vi "Configure FFT.vi"(7 "FFT Parameters":T2={"Direction"=TRUE, "scale_sch"=85.0, "Flush Length"=1500} {"scale_sch" format="%.0b"}, 8 "error in":errorcluster, 11 "FPGA Session":T1) -> (0 "error out":errorcluster, 3 "FPGA Session":T1)   [LabVIEW 2010]
doc: "This VI configures FFT Length, Scaling Parameters from the Host.\n\nThis VI also starts FFT Core on the FPGA and waits for valid input to start processing data."
uses:
  Session/Session Handle.ctl
  FFT Block/FFT/Controls/FFT Parameters.ctl
  <vilib>/rvi/interface/nirviReadWriteControl/nirviReadWriteControl.xnode
  System Integration Test Bench/tb_Interpolate and FFT Loop/tb_interpolation_fft_simio_fpga.vi
  FFT Block/FFT/Controls/FFT States.ctl
  <vilib>/RVI Host/nirviSupport.llb/nirviErrorClusterFromErrorCode.vi
  <vilib>/rvi/errors/niLvFpgaWhatHappensToTopLevelVI.ctl
  <vilib>/rvi/interface/common/niFpgaNodeNameForErrorReporting.ctl
  <vilib>/rvi/errors/niLvFpgaAdjustHostInterfaceError.vi
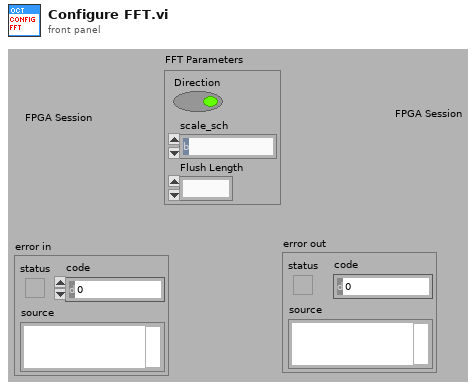
[diagram p1: front panel]
types:
  T1 = typedef "Session Handle.ctl" = refnum<k20>
  T2 = typedef "FFT Parameters.ctl" = cluster{"Direction":bool, "scale_sch":fxp<+,10,10>, "Flush Length":u16}
  T3 = typedef "FFT States.ctl" = enum8{"Configure", "Start FFT processing", "Process", "Unload Last FFT", "Reset"}
  T4 = typedef "niFpgaNodeNameForErrorReporting.ctl" = enum16{"Open FPGA VI Reference", "Read/Write Control", "Invoke Method: Abort", "Invoke Method: Acknowledge IRQ", "Invoke Method: Download", "Invoke Method: FIFO.Configure", "Invoke Method: FIFO.Read", "Invoke Method: FIFO.Start", "Invoke Method: FIFO.Stop", "Invoke Method: FIFO.Write", "Invoke Method: Reset", "Invoke Method: Run", "Invoke Method: Wait on IRQ", "Close FPGA VI Reference"}
  T5 = typedef "niLvFpgaWhatHappensToTopLevelVI.ctl" = enum16{"top level VI scripted behind XNode", "top level VI inlined behind XNode"}
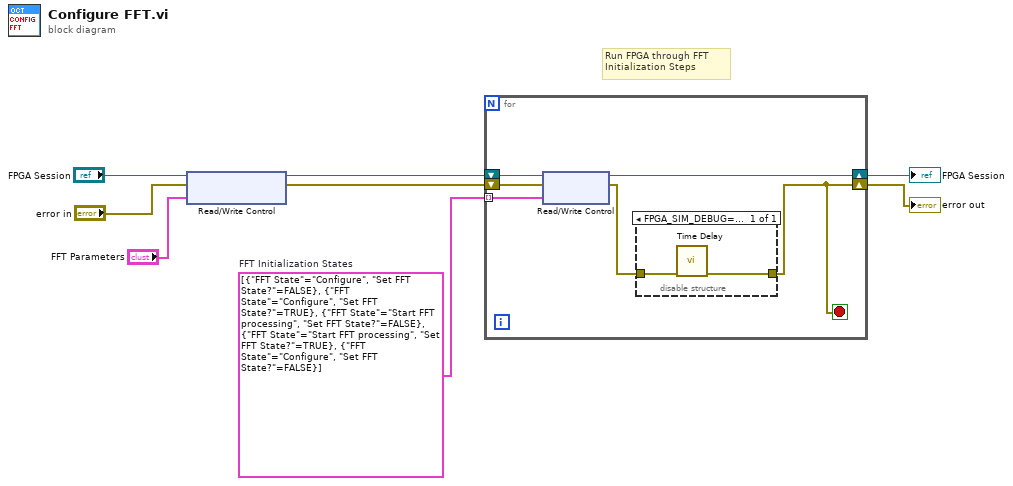
[diagram p0: block diagram]
diagram:
  w3 = cluster{"FFT State":T3, "Set FFT State?":bool}[] [{"FFT State"=enum."Configure", "Set FFT State?"=FALSE}, {"FFT State"=enum."Configure", "Set FFT State?"=TRUE}, {"FFT State"=enum."Start FFT processing", "Set FFT State?"=FALSE}, {"FFT State"=enum."Start FFT processing", "Set FFT State?"=TRUE}, {"FFT State"=enum."Configure", "Set FFT State?"=FALSE}]  # FFT Initialization States
  # "Run FPGA through FFT \nInitialization Steps"
  n1 = xnode "Read/Write Control"("FPGA VI Reference In"="FPGA Session", "error in"="error in", "FFT Parameters"="FFT Parameters") -> ("FPGA VI Reference Out"=w8:T1, "error out"=w7:errorcluster)
  n2 = for {
    shift-right: [w12] -> w2
    shift-left: w8 -> [w14]
    shift-right: [w9] -> w1
    shift-left: w7 -> [w13]
    tunnel: w3 -> [w11] mode=indexing
    stop <- w9 stop-if-true
    n3 = xnode "Read/Write Control"("FPGA VI Reference In"=w14, "error in"=w13, "FFT State"=w11) -> ("FPGA VI Reference Out"=w12:T1, "error out"=w10:errorcluster)
    n4 = disable-structure shown="FPGA_SIM_DEBUG==TRUE, default" {
      disable-tunnel: w10 -> [w16]
      disable-tunnel: [w15] -> w9
      frame condition #0 (active) {
        n5 = call "Time Delay"("error in (no error)"=w16) -> ("error out"=w15:errorcluster)  [unwired: 10 in]
      }
    }
  }
  "error out" <- w1
  "FPGA Session" <- w2
